vi "Last Ack.vi"(7 "Is Sync":bool, 10 "Actor":refnum<class "Actor.lvclass">) -> (2 "Msg":refnum<class "Msg.lvclass">)   [LabVIEW 2021, in "jettl.lvlib" / "Last Ack Msg.lvlib"]
uses:
  Last Ack Msg.lvlib
  Msg/Msg.lvclass
  Actor/Actor/Actor.lvclass
  Last Ack Msg/Last Ack Msg.lvclass
  C:/git/jettl/jettl/jettl/Msg/Msg.lvclass
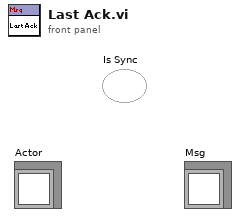
[diagram p1: front panel]
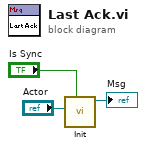
[diagram p0: block diagram]
diagram:
  n1 = call "Init.vi"("Is Sync"="Is Sync", "Actor"="Actor") -> ("Last Ack Msg out"=→"Msg":refnum<class "Last Ack Msg.lvclass">)  [unwired: 9 in]
